vi "Meas Freq of Visible Waveform LV 2012.vi"(8 "error in":errorcluster, 11 "Waveform Graph Reference":refnum<vi>) -> (0 "error out":errorcluster, 2 "Frequency":dbl, 3 "Waveform Graph Reference Out":refnum<vi>)   [LabVIEW 2015]
uses:
  <vilib>/Analysis/NI_AALBase.lvlib
  <vilib>/Analysis/baseanly.llb/Mean (DBL).vi
panel:
  in  "waveform":waveform(dbl)={"t0"=timestamp(0 s since 1904-01-01), "dt"=0.0, "Y"=[]}
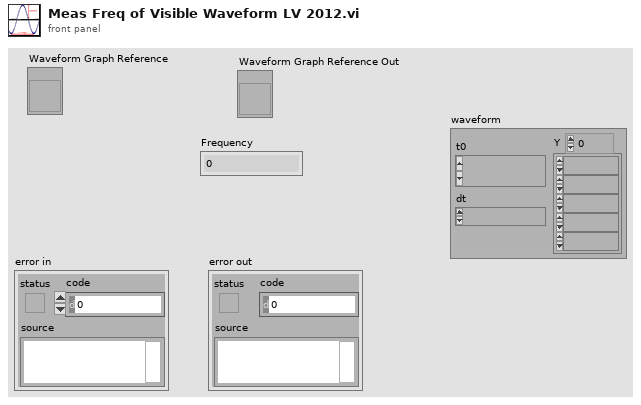
[diagram p1: front panel]
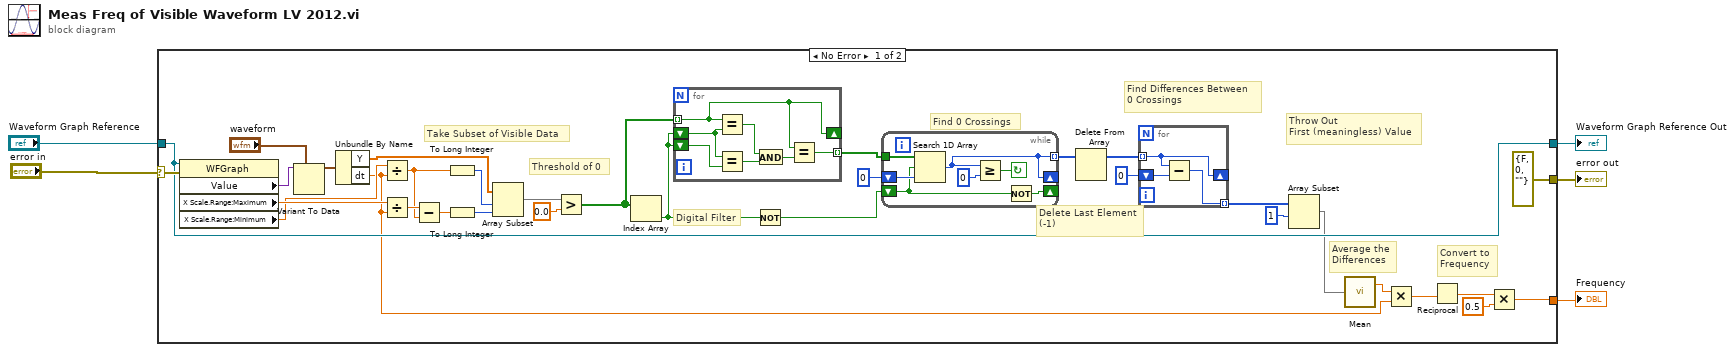
[diagram p0: block diagram]
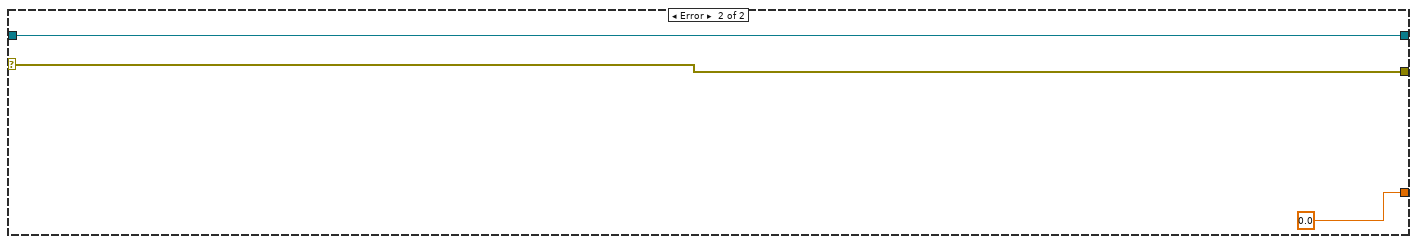
[diagram p2: hidden frame]
diagram:
  n1 = case shown="No Error" "error in" {
    selector: "error in" -> [w38 w58]
    tunnel: [w17 0.0] -> w5
    tunnel: "Waveform Graph Reference" -> [w36 w56]
    tunnel: [errorcluster {"status"=FALSE, "code"=0, "source"=""} ("error IO") w58] -> w2
    tunnel: [w36 w56] -> w1
    frame No Error {
      # "Delete Last Element\n(-1)"
      # "Convert to\nFrequency"
      # "Average the\nDifferences"
      # "Take Subset of Visible Data"
      # "Throw Out\nFirst (meaningless) Value"
      # "Find Differences Between\n0 Crossings"
      # "Threshold of 0"
      # "Find 0 Crossings"
      # "Digital Filter"
      n2 = property on="Property Node" class="WFGraph"(reference=w36, error in=w38) -> ("Value"=w10:variant, "X Scale.Range:Maximum"=w28:dbl, "X Scale.Range:Minimum"=w27:dbl)  [unwired: 2 out]
      n3 = Variant To Data(type="waveform", Variant=w10) -> (data=w9:waveform(dbl))  [unwired: 1 in, 1 out]
      n4 = Unbundle By Name(w9) -> ("Y"=w29:dbl[], "dt"=w21:dbl)
      n5 = Divide(x=w27, y=w21) -> (x/y=w23:dbl)
      n6 = Divide(x=w28, y=w21) -> (x/y=w26:dbl)
      n7 = Subtract(x=w26, y=w23) -> (x-y=w25:dbl)
      n8 = To Long Integer(number=w23) -> (32bit integer=w22:i32)
      n9 = To Long Integer(number=w25) -> (32bit integer=w24:i32)
      n10 = Array Subset(array=w29, index=w22, length=w24) -> (w13:dbl[])
      n11 = Greater?(x=w13, y=0.0) -> (0:w33:bool[])
      n12 = Index Array(array=w33) -> (element=w12:bool)  [unwired: 1 in]
      n13 = for {
        tunnel: w33 -> [w50] mode=indexing
        shift-right: [w50] -> _
        shift-left: w12 -> [w55]
        shift-left: w12 -> [w54]
        tunnel: [w49] -> w16 mode=indexing
        n14 = Equal?(x=w50, y=w55) -> (x = y?=w53:bool)
        n15 = Equal?(x=w55, y=w54) -> (x = y?=w52:bool)
        n16 = And(x=w53, y=w52) -> (x .and. y?=w51:bool)
        n17 = Equal?(x=w50, y=w51) -> (x = y?=w49:bool)
      }
      n18 = Not(x=w12) -> (.not. x?=w11:bool)
      n19 = while {
        tunnel: w16 -> [w48]
        shift-right: [w44] -> _
        shift-left: 0 ("index of element") -> [w47]
        tunnel: [w44] -> w15 mode=indexing
        shift-right: [w46] -> _
        shift-left: w11 -> [w45]
        stop <- w42 continue-if-true
        n20 = Search 1D Array(1D array=w48, element=w45, start index (0)=w47) -> (index of element=w44:i32)
        n21 = Greater Or Equal?(x=w44, y=0) -> (x >= y?=w42:bool)
        n22 = Not(x=w45) -> (.not. x?=w46:bool)
      }
      n23 = Delete From Array(array=w15) -> (array with subset deleted=w14:i32[])  [unwired: 2 in, 1 out]
      n24 = for {
        tunnel: w14 -> [w41] mode=indexing
        shift-right: [w41] -> _
        shift-left: 0 ("index of element") -> [w40]
        tunnel: [w39] -> w32 mode=indexing
        n25 = Subtract(x=w41, y=w40) -> (x-y=w39:i32)
      }
      n26 = Array Subset(array=w32, index=1) -> (w7:i32[])  [unwired: 1 in]
      n27 = call-poly <vilib>:"Mean.vi"("X"=w7) -> ("mean"=w6:dbl)  [unwired: 1 out]
      n28 = Multiply(x=w6, y=w21) -> (x*y=w20:dbl)
      n29 = Reciprocal(x=w20) -> (1/x=w19:dbl)
      n30 = Multiply(x=w19, y=0.5) -> (x*y=w17:dbl)
    }
    frame Error {
    }
  }
  "Frequency" <- w5
  "error out" <- w2
  "Waveform Graph Reference Out" <- w1
